vi "DisposeImage.vi"(8 "error in (no error)":errorcluster, 11 "Image in":refnum<k24>) -> (0 "error out":errorcluster)   [LabVIEW 2020, in "FaceRecognitionDotNet.lvlib" / "FaceRecognition.lvclass"]
uses:
  FaceRecognition.lvclass
  dll/FaceRecognitionDotNet.dll
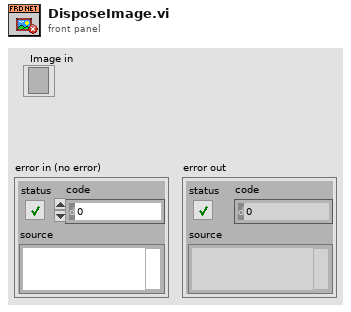
[diagram p1: front panel]
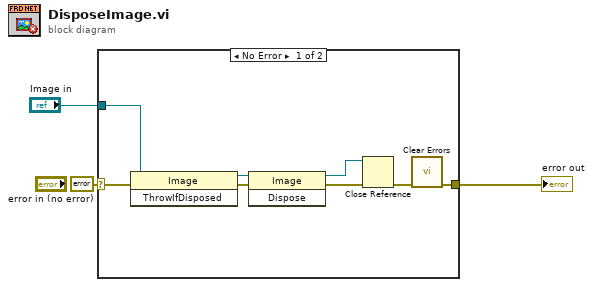
[diagram p0: block diagram]
diagram:
  n1 = case shown="No Error" errorcluster {"status"=FALSE, "code"=0, "source"=""} ("error IO") {
    selector: errorcluster {"status"=FALSE, "code"=0, "source"=""} ("error IO") -> [w7 w12]
    tunnel: "Image in" -> [w9 _]
    tunnel: [w8 w12] -> w2
    frame No Error {
      n2 = invoke class="Image" method="ThrowIfDisposed"(reference=w9, error in=w7) -> (reference out=w10:refnum<k24>, error out=w11:errorcluster)  [unwired: 1 in, 1 out]
      n3 = invoke class="Image" method="Dispose"(reference=w10, error in=w11) -> (reference out=w6:refnum<k24>, error out=w5:errorcluster)  [unwired: 1 in, 1 out]
      n4 = Close Reference(reference=w6, error in (no error)=w5) -> (error out=w4:errorcluster)
      n5 = call <vilib>:"Clear Errors.vi"("error in (no error)"=w4) -> ("error out"=w8:errorcluster)  [unwired: 5 in, 1 out]
    }
    frame Error {
    }
  }
  "error out" <- w2
